vi "calcStartPos.vi"(0 "Measured origin x,y":dbl[](array[numeric]), 1 "Origin to jet outlet (Jet toal)":dbl, 2 "Numeric":dbl, 3 "Hight to groove(tube center)":dbl, 4 "a0 radius":dbl) -> (5 "Array":dbl[](array[numeric]))   [LabVIEW 2009]
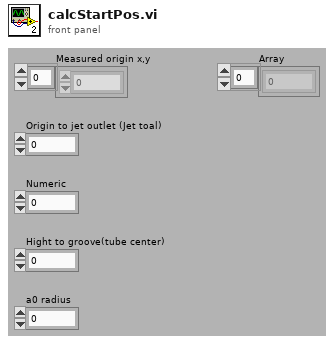
[diagram p1: front panel]
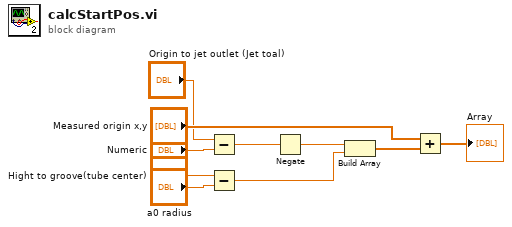
[diagram p0: block diagram]
diagram:
  n1 = Subtract(x="Origin to jet outlet (Jet toal)", y="Numeric") -> (x-y=w3:dbl)
  n2 = Subtract(x="Hight to groove(tube center)", y="a0 radius") -> (x-y=w7:dbl)
  n3 = Negate(x=w3) -> (-x=w6:dbl)
  n4 = Build Array(w6, w7) -> (w9:dbl[])
  n5 = Add(x="Measured origin x,y", y=w9) -> (x+y=→"Array":dbl[])
